vi "Set APU&ECU Cntrls.vi"(8 "error in (no error)":errorcluster, 11 "APU & ECU Controls":T1) -> (0 "error out":errorcluster)   [LabVIEW 2018, in "Outputs.lvlib"]
doc: "This subVI enqueues the named action in to the communications queue along with the input data."
uses:
  Outputs.lvlib
  Modules/Testing UI 1/Private Controls/APU & ECU Controls.ctl
  Private Controls/Module Data.ctl
  Private Controls/Module Action.ctl
  Modules/Testing UI 1/Testing UI 1.lvlib
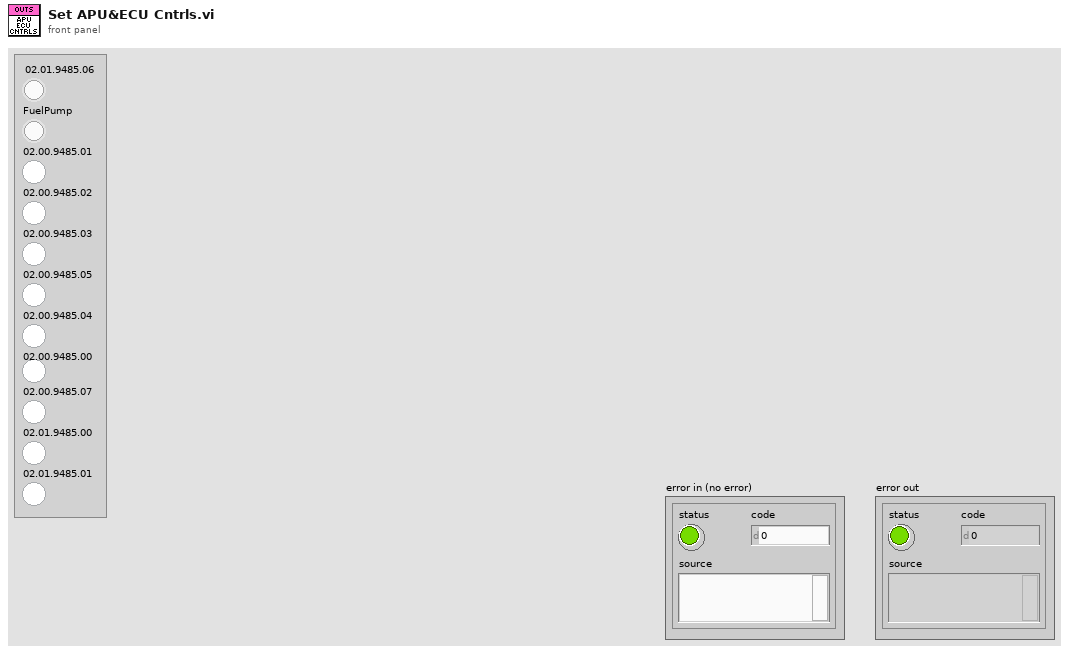
[diagram p1: front panel]
types:
  T1 = typedef "Testing UI 1.lvlib/APU & ECU Controls.ctl" = cluster{"02.01.9485.06":bool, "FuelPump":bool, "02.00.9485.01":bool, "02.00.9485.02":bool, "02.00.9485.03":bool, "02.00.9485.05":bool, "02.00.9485.04":bool, "02.00.9485.00":bool, "02.00.9485.07":bool, "02.01.9485.00":bool, "02.01.9485.01":bool}
  T2 = typedef "Outputs.lvlib/Module Data.ctl" = cluster{"Data":variant, "Action":T3}
  T3 = typedef "Outputs.lvlib/Module Action.ctl" = enum16{"Init", "Error", "Write 02-06-9265 Vals (AO)", "Write 02-01-9485 Vals (DO)", "Set APU&ECU Cntrls", "Set Bleed-Fuel-ECS Cntrls", "Set ECS Demnd Cluster", "Set Fuel Pres Regltr", "Write Single 02-00-9485 Chann", "Write Single 02-01-9485 Chann"}
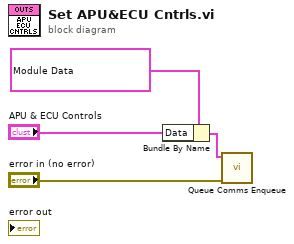
[diagram p0: block diagram]
diagram:
  n1 = Bundle By Name(cluster=T2 {"Data"=variant, "Action"=enum."Set APU&ECU Cntrls"} ("element"), "Data"="APU & ECU Controls") -> (w3:T2)
  n2 = call "Queue Comms Enqueue.vi"("error in (no error)"="error in (no error)", "element"=w3) -> ()  [unwired: 9 in, 1 out]
